vi "Formating And Concatenate Strings.vi"() -> ()   [LabVIEW 2012]
panel:
  out "Date/Time + Output String In Correct Format":string
  in  "Input String":string="Hello World"
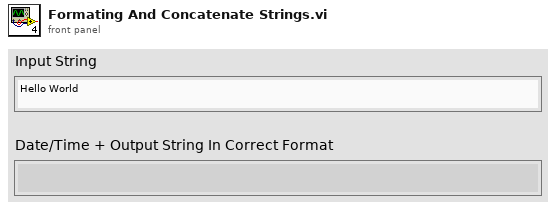
[diagram p1: front panel]
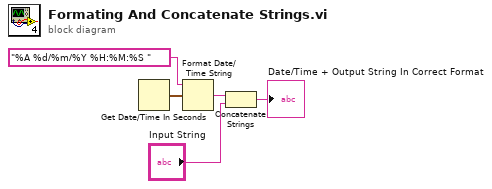
[diagram p0: block diagram]
diagram:
  n1 = Get Date/Time In Seconds() -> (seconds since 1Jan1904=w5:timestamp)
  n2 = Format Date/Time String(time format string (%c)="%A %d/%m/%Y %H:%M:%S ", seconds (now)=w5) -> (date/time string=w4:string)  [unwired: 1 in]
  n3 = Concatenate Strings(w4, "Input String") -> (→"Date/Time + Output String In Correct Format":string)
